vi "Detect_Pulses.vi"(8 "error in (no error)":errorcluster, 9 "threshold":dbl, 10 "Y":dbl[](array[numeric]), 11 "dt":dbl) -> (0 "error out":errorcluster, 1 "Locations":dbl[](array[numeric]), 2 "# found":i32, 3 "Waveform":waveform(dbl), 5 "Amplitudes":dbl[](array[numeric]))   [LabVIEW 2020]
uses:
  <vilib>/measure/mamon.llb/Waveform Peak Detection for 1 Chan.vi
  <vilib>/measure/NI_MAPro.lvlib
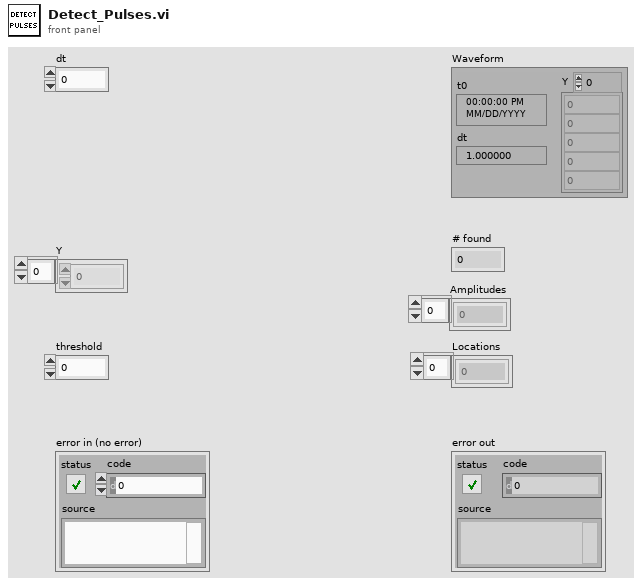
[diagram p1: front panel]
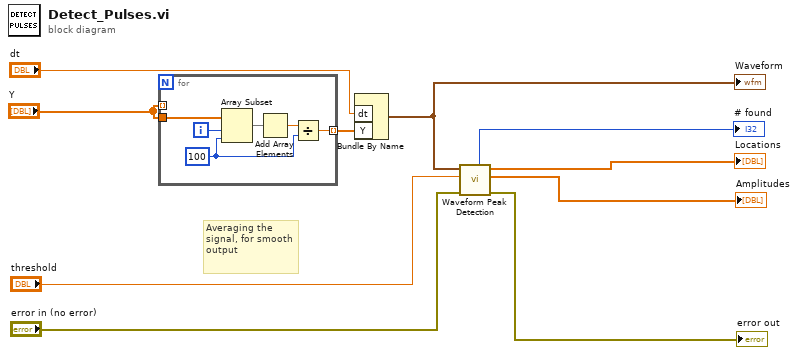
[diagram p0: block diagram]
diagram:
  # "Averaging the signal, for smooth output"
  n1 = for {
    tunnel: "Y" -> [_] mode=indexing
    tunnel: "Y" -> [w15]
    tunnel: [w11] -> w2 mode=indexing
    i -> [w16]
    w12 = 100 ("length")
    n2 = Array Subset(array=w15, index=w16, length=w12) -> (w14:dbl[])
    n3 = Add Array Elements(numeric array=w14) -> (sum=w13:dbl)
    n4 = Divide(x=w13, y=w12) -> (x/y=w11:dbl)
  }
  n5 = Bundle By Name("dt"="dt", "Y"=w2) -> (w4:waveform(dbl))  [unwired: 1 in]
  "Waveform" <- w4
  n6 = call-poly <vilib>:"Waveform Peak Detection.vi"("error in"="error in (no error)", "threshold"="threshold", "Signal In"=w4) -> ("error out"=→"error out":errorcluster, "Amplitudes"=→"Amplitudes":dbl[], "Locations"=→"Locations":dbl[], "# found"=→"# found":i32)  [unwired: 4 in, 1 out]
